vi "constructor.vi"(8 "error in (no error)":errorcluster, 11 "deviceName":string) -> (0 "error out":errorcluster, 3 "DigitalOutput out":refnum<class "DigitalOutput.lvclass">)   [LabVIEW 2011, in "Hardware.lvlib" / "Channels.lvlib" / "DigitalOutput.lvclass"]
uses:
  DigitalOutput.lvclass
  DIO64Output.lvclass
  niDAQmxDO.lvclass
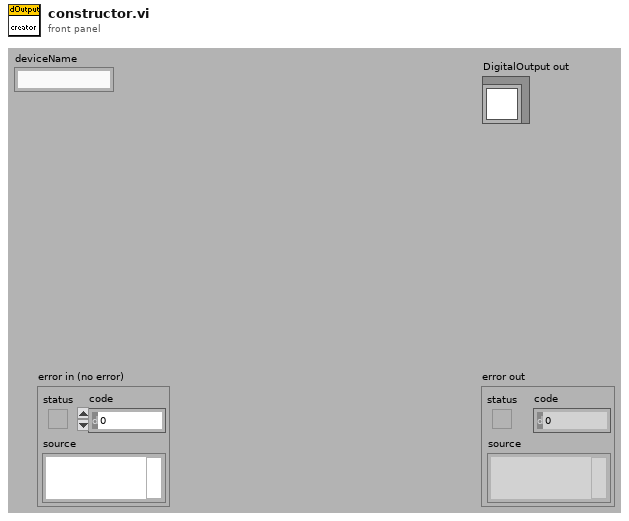
[diagram p1: front panel]
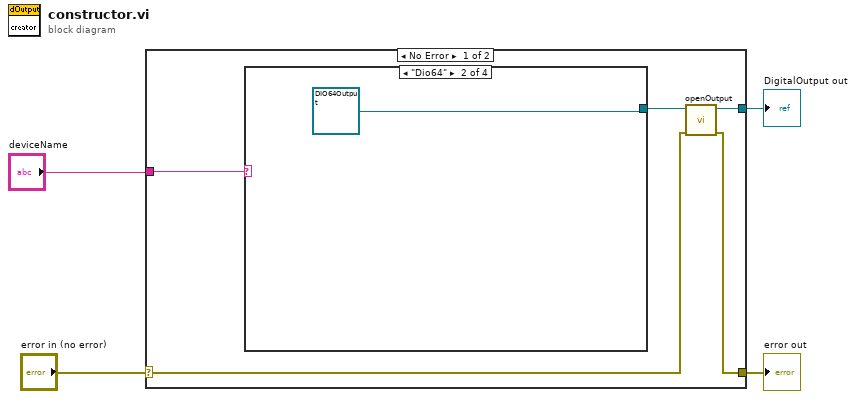
[diagram p0: block diagram]
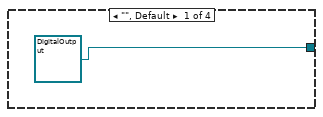
[diagram p2: hidden frame]
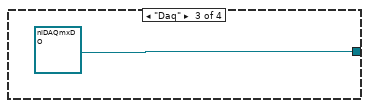
[diagram p3: hidden frame]
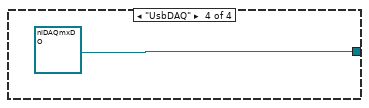
[diagram p4: hidden frame]
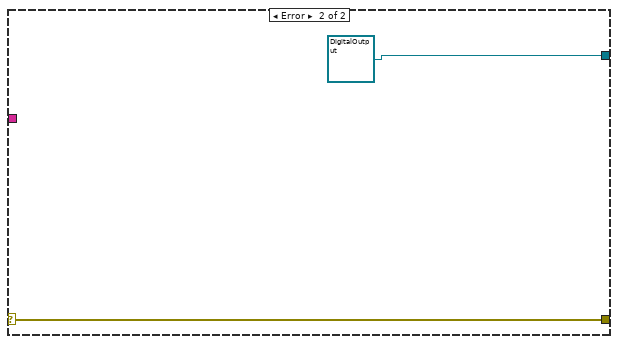
[diagram p5: hidden frame]
diagram:
  n1 = case shown="No Error" "error in (no error)" {
    selector: "error in (no error)" -> [w5 w15]
    tunnel: [w6 w15] -> w3
    tunnel: [w7 refnum<class "DigitalOutput.lvclass"> refnum ("Hardware:Channels.lvlib:DigitalOutput.lvclass")] -> w2
    tunnel: "deviceName" -> [w9 _]
    frame No Error {
      n2 = case shown="\"Dio64\"" w9 {
        tunnel: [refnum<class "DigitalOutput.lvclass"> refnum ("Hardware:Channels.lvlib:DigitalOutput.lvclass") refnum<class "DIO64Output.lvclass"> refnum ("Hardware:Channels.lvlib:DIO64Output.lvclass") refnum<class "niDAQmxDO.lvclass"> refnum ("Hardware:Channels.lvlib:niDAQmxDO.lvclass") refnum<class "niDAQmxDO.lvclass"> refnum ("Hardware:Channels.lvlib:niDAQmxDO.lvclass")] -> w8
        frame "", Default {
        }
        frame "Dio64" {
        }
        frame "Daq" {
        }
        frame "UsbDAQ" {
        }
      }
      n3 = call-dynamic "openOutput.vi"("error in (no error)"=w5, "DigitalOutput in"=w8) -> ("error out"=w6:errorcluster, "DigitalOutput out"=w7:refnum<class "DigitalOutput.lvclass">)  [unwired: 8 in]
    }
    frame Error {
    }
  }
  "error out" <- w3
  "DigitalOutput out" <- w2
